vi "Variable dispatch.vi"() -> ()   [LabVIEW 2020, in "Library Instrument & Equipement.lvlib" / "Process (Default).lvclass"]
uses:
  Process (Default).lvclass
panel:
  in  "Ref_HMI":refnum<vi>
  in  "Class Process":refnum<class "Process (Default).lvclass">
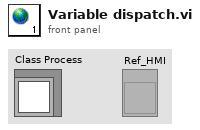
[diagram p1: front panel]
diagram:
